vi "signal input-A.vi"(8 "Reference Signal":cluster{dbl[], dbl[]}, 9 "Coherent Noise":cluster{"F":dbl, "Ampl":dbl}[](array[cluster]), 10 "Time":dbl, 11 "Input":T1 {"AM Frequency" format="%.4f"; "AM Amplitude" format="%.4f"; "LOCK-IN Freq" format="%.2f"; "LOCK-IN Phase" format="%.2f"; "Time Constant (sec)" format="%.2f"; "Low-pass filter slope" format="%.2f"; "Spectral Amplitude" format="%.2f"; "Phase Angle" scale=0.0..360.0 scale format="%.1f"; "Frequency" format="%.2f"; "Amplitude" format="%.2f"}) -> (3 "OUTPUT":T2 {"Input Signal" format="%.2f"; "LOCK-IN Freq" format="%.2f"; "LOCK-IN Phase" format="%.2f"; "Time Constant (sec)" format="%.2f"; "Low-pass filter scope" format="%.2f"; "Time" format="%.2f"; "Spectral Amplitude" format="%.2f"; "Phase Angle" format="%.2f"; "Frequency" format="%.2f"; "Amplitude" format="%.2f"})   [LabVIEW 2023]
doc: "This VI generates the input signal for the Lock-In, starting at TIME. COHERENT NOISE can also be added."
uses:
  <vilib>/ptbypt/NI_PtbyPt.lvlib
panel:
  in  "Beta":dbl
  in  "fm [Hz]":dbl
  out "Waveform Chart":cluster{"sine wave":dbl, dbl}(graph)
  out "Signal w/ noise":dbl format="%.2f"
  out "Pure Signal":dbl format="%.2f"
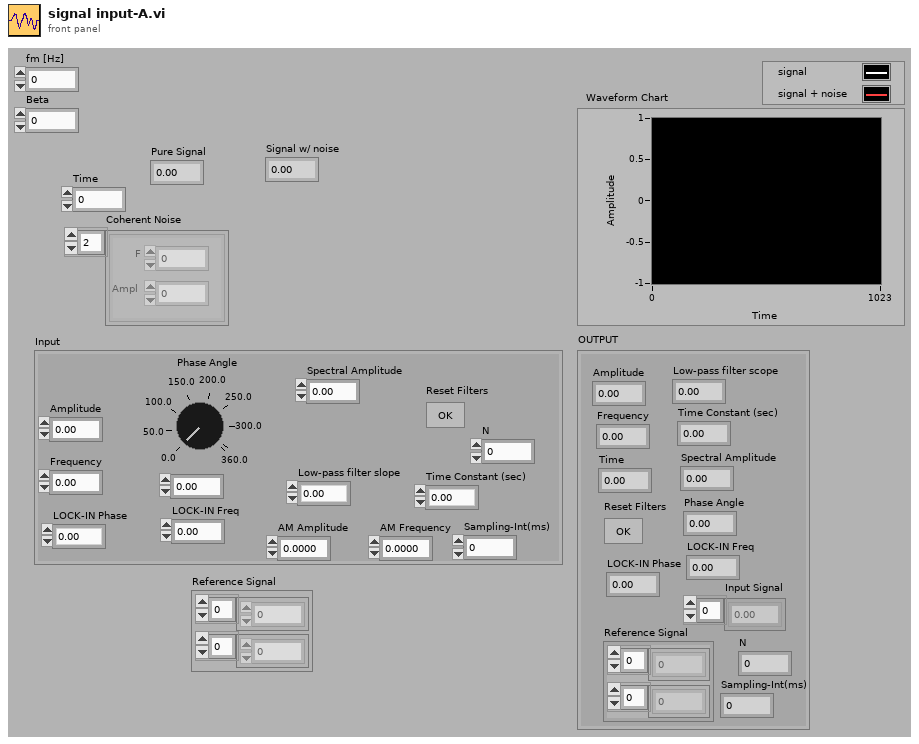
[diagram p1: front panel]
types:
  T1 = cluster{"Amplitude":dbl, "Frequency":dbl, "Phase Angle":dbl, "Spectral Amplitude":dbl, "Low-pass filter slope":dbl, "Time Constant (sec)":dbl, "Reset Filters":bool, "LOCK-IN Phase":dbl, "LOCK-IN Freq":dbl, "AM Amplitude":dbl, "AM Frequency":dbl, "Sampling-Int(ms)":dbl, "N":i32}
  T2 = cluster{"Amplitude":dbl, "Frequency":dbl, "Phase Angle":dbl, "Spectral Amplitude":dbl, "Time":dbl, "Low-pass filter scope":dbl, "Time Constant (sec)":dbl, "Reset Filters":bool, "LOCK-IN Phase":dbl, "LOCK-IN Freq":dbl, "Sampling-Int(ms)":dbl, "Reference Signal":cluster{dbl[], dbl[]}, "Input Signal":dbl[], "N":i32}
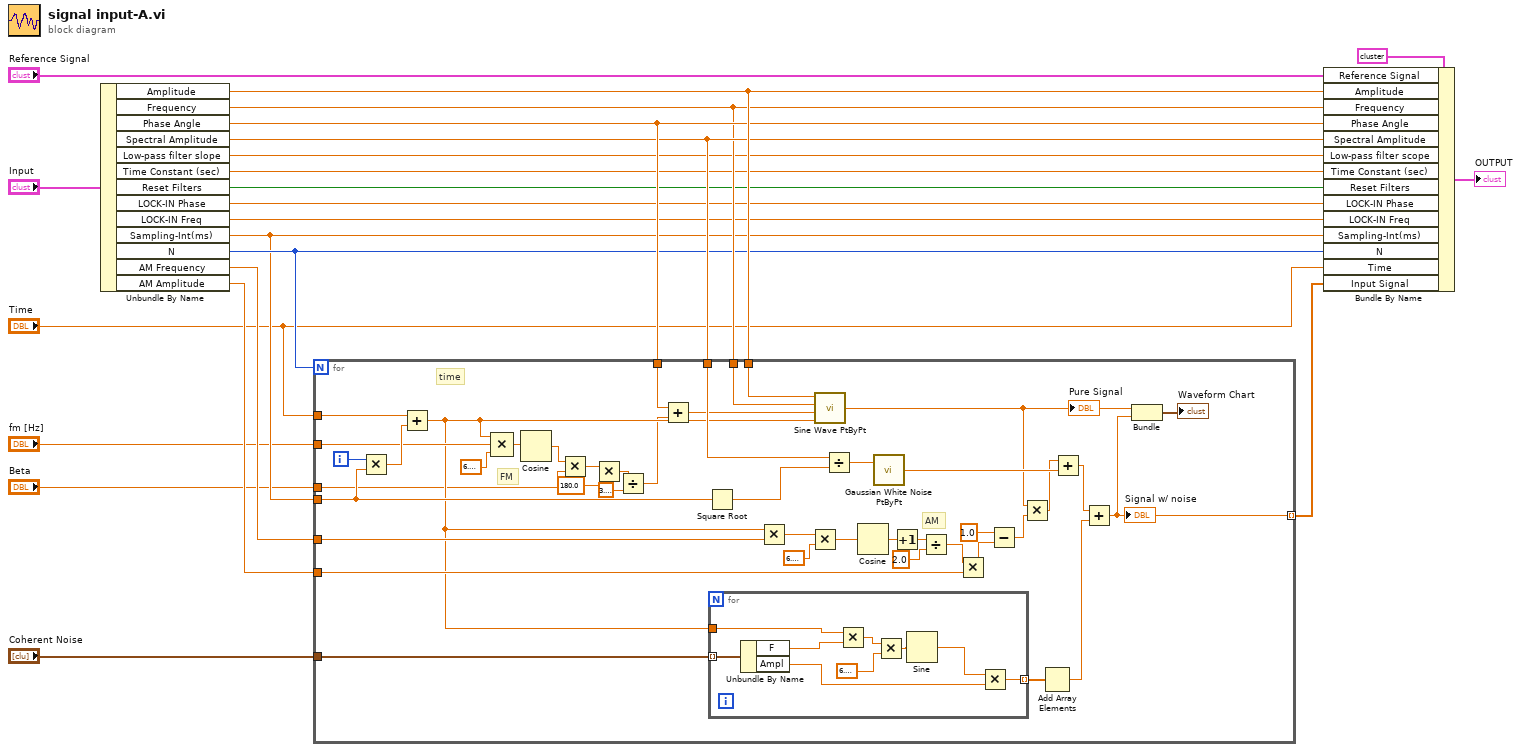
[diagram p0: block diagram]
diagram:
  n1 = Unbundle By Name("Input") -> ("Amplitude"=w22:dbl, "Frequency"=w17:dbl, "Phase Angle"=w21:dbl, "Spectral Amplitude"=w20:dbl, "Low-pass filter slope"=w16:dbl, "Time Constant (sec)"=w15:dbl, "Reset Filters"=w14:bool, "LOCK-IN Phase"=w13:dbl, "LOCK-IN Freq"=w12:dbl, "Sampling-Int(ms)"=w8:dbl, "N"=w9:i32, "AM Frequency"=w6:dbl, "AM Amplitude"=w4:dbl)
  n2 = for {
    N: w9 -> [_]
    tunnel: w22 -> [w65]
    tunnel: w17 -> [w64]
    tunnel: w21 -> [w33]
    tunnel: w20 -> [w55]
    tunnel: "Time" -> [w59]
    tunnel: w6 -> [w62]
    tunnel: w4 -> [w61]
    tunnel: [w40] -> w5 mode=indexing
    tunnel: w8 -> [w48]
    tunnel: "Coherent Noise" -> [w49]
    tunnel: "fm [Hz]" -> [w36]
    tunnel: "Beta" -> [w31]
    i -> [w60]
    # "AM"
    # "FM"
    # "time"
    n3 = Multiply(x=w60, y=w48) -> (x*y=w58:dbl)
    n4 = Add(x=w59, y=w58) -> (x+y=w35:dbl)
    n5 = Compound Arithmetic op=MULTIPLY(w35, w36, 6.283185307179586) -> (w38:dbl)
    n6 = Cosine(x=w38) -> (cos(x)=w32:dbl)
    n7 = Multiply(x=w32, y=w31) -> (x*y=w27:dbl)
    n8 = Multiply(x=w27, y=180.0) -> (x*y=w26:dbl)
    n9 = Divide(x=w26, y=3.141592653589793) -> (x/y=w24:dbl)
    n10 = Add(x=w33, y=w24) -> (x+y=w34:dbl)
    n11 = Square Root(x=w48) -> (sqrt(x)=w54:dbl)
    n12 = for {
      tunnel: w49 -> [w74] mode=indexing
      tunnel: [w72] -> w53 mode=indexing
      tunnel: w35 -> [w67]
      n13 = Unbundle By Name(w74) -> ("F"=w69:dbl, "Ampl"=w73:dbl)
      n14 = Multiply(x=w67, y=w69) -> (x*y=w71:dbl)
      n15 = Multiply(x=w71, y=6.283185307179586) -> (x*y=w70:dbl)
      n16 = Sine(x=w70) -> (sin(x)=w66:dbl)
      n17 = Multiply(x=w66, y=w73) -> (x*y=w72:dbl)
    }
    n18 = Multiply(x=w35, y=w62) -> (x*y=w51:dbl)
    n19 = Multiply(x=w51, y=6.283185307179586) -> (x*y=w50:dbl)
    n20 = call <vilib>:"Sine Wave PtByPt.vi"("time"=w35, "phase"=w34, "frequency"=w64, "amplitude"=w65) -> ("sine wave"=w37:dbl)
    "Pure Signal" <- w37
    n21 = Divide(x=w55, y=w54) -> (x/y=w56:dbl)
    n22 = Cosine(x=w50) -> (cos(x)=w44:dbl)
    n23 = call <vilib>:"Gaussian White Noise PtByPt.vi"("standard deviation"=w56) -> ("Gaussian white noise"=w63:dbl)  [unwired: 2 in]
    n24 = Increment(x=w44) -> (x+1=w43:dbl)
    n25 = Divide(x=w43, y=2.0) -> (x/y=w42:dbl)
    n26 = Multiply(x=w42, y=w61) -> (x*y=w46:dbl)
    n27 = Subtract(x=1.0, y=w46) -> (x-y=w45:dbl)
    n28 = Multiply(x=w37, y=w45) -> (x*y=w30:dbl)
    n29 = Add Array Elements(numeric array=w53) -> (sum=w28:dbl)
    n30 = Add(x=w30, y=w63) -> (x+y=w29:dbl)
    n31 = Add(x=w29, y=w28) -> (x+y=w40:dbl)
    "Signal w/ noise" <- w40
    n32 = Bundle("sine wave"=w37, w40) -> (→"Waveform Chart":cluster{"sine wave":dbl, dbl})  [unwired: 1 in]
  }
  n33 = Bundle By Name(cluster=T2 {"Amplitude"=1.0, "Frequency"=90.0, "Phase Angle"=0.0, "Spectral Amplitude"=3.1622776601683794e-12, "Time"=15.5, "Low-pass filter scope"=2.0, "Time Constant (sec)"=3.0, "Reset Filters"=TRUE, "LOCK-IN Phase"=0.0, "LOCK-IN Freq"=90.0, "Sampling-Int(ms)"=0.001, "Reference Signal"={array[100000 elements], array[100000 elements]}, "Input Signal"=[3.6270014704731955e-10, 0.7639707479411351, 0.32806858266099154, 0.03116910771588919, 0.6261334584508225, 0.559016994196243, -0.46661849662936283, -0.683196308630999, -0.06897966261191531, -0.25199859719526513, -0.7694208844477284, -0.1250859172372213, 0.7398902012390709, 0.4067580802859709, 0.007869738850446182, 0.5590169943230116, 0.6364758026279465, -0.3616040548870293, -0.7275301742948549, -0.11980726686689382, -0.1816356320077278, -0.7568653348095259, -0.24672889297442516, 0.697181226573696, 0.48483057948780817, 0.0, 0.48483057963293147, 0.6971812260973207, -0.24672889332109527, -0.7568653348144952, -0.18163563204574137, -0.1198072668350432, -0.7275301744952588, -0.3616040548022246, 0.6364758024591584, 0.5590169943173463, 0.00786973885047025, 0.40675808032800603, 0.7398902013892035, -0.12508591739506292, -0.769420884183334, -0.25199859714365924, -0.06897966261341107, -0.6831963085445812, -0.46661849653327014, 0.5590169940952557, 0.6261334586645678, 0.031169107708940127, 0.32806858266562805, 0.7639707483194247, 3.050194502447735e-10, -0.7639707481316645, -0.3280685826235266, -0.03116910771200357, -0.6261334583012064, -0.5590169945442752, 0.46661849661387955, 0.6831963086207411, 0.06897966261637724, 0.251998597161211, 0.7694208845491353, 0.12508591737979402, -0.7398902015961744, -0.40675808019389864, -0.00786973884866858, -0.5590169943866681, -0.6364758029756332, 0.3616040547369034, 0.7275301742380216, 0.11980726683753752, 0.18163563197239485, 0.7568653349769223, 0.24672889325318684, -0.6971812263598314, -0.4848305795125243, 0.0, -0.4848305794652994, -0.6971812262925658, 0.24672889337578283, 0.7568653350268335, 0.18163563201669025, 0.11980726684926235, 0.727530174431457, 0.36160405447869354, -0.6364758024685663, -0.5590169942792828, -0.007869738852104208, -0.40675808027683447, -0.7398902012745293, 0.1250859170488911, 0.7694208841740288, 0.2519985971529551, 0.0689796626074951, 0.6831963086494821, 0.46661849653975535, -0.5590169941653226, -0.6261334584911336, -0.031169107715581835, -0.32806858260126787, -0.7639707482084847], "N"=100} ("OUTPUT"), "Reference Signal"="Reference Signal", "Amplitude"=w22, "Frequency"=w17, "Phase Angle"=w21, "Spectral Amplitude"=w20, "Low-pass filter scope"=w16, "Time Constant (sec)"=w15, "Reset Filters"=w14, "LOCK-IN Phase"=w13, "LOCK-IN Freq"=w12, "Sampling-Int(ms)"=w8, "N"=w9, "Time"="Time", "Input Signal"=w5) -> (→"OUTPUT":T2)
